vi "DataLog Logging Module.vi"(5 "LuaVIEW reference":T2, 7 "function index":i32) -> (15 "error out":errorcluster)   [LabVIEW 2012]
doc: "Modules required by the \"datalogging\" runlevel. It initializes the logging objects required when the current database goes live. It also exports functions for monitoring and influencing the logging."
uses:
  luaview/typedefs/t_LuaVIEW Reference.ctl
  typedefs/t_DataLog Tag Meta Tags Methods.ctl
  typedefs/t_DataLog Tag Buffers Methods.ctl
  typedefs/t_DataLog Tag Info List Methods.ctl
  typedefs/t_DataLog Live Tag Strings Methods.ctl
  typedefs/t_DataLog Tag Hash Methods.ctl
  typedefs/t_DataLog Aggregation Buffer Methods.ctl
  typedefs/t_DataLog Tag Expression Evaluator Methods.ctl
  luaview/subvis/private/LuaVIEW Pull (string).vi
  luaview/subvis/private/LuaVIEW Pull (refnum).vi
  luaview/subvis/private/LuaVIEW Pull (flat data).vi
  subvis/private/glb_DataLog Runtime Parameterisation.vi
  luaview/subvis/private/LuaVIEW Push (boolean).vi
  luaview/subvis/private/LuaVIEW Push (number).vi
panel:
  in  "config":T1={"aggregation capacity"=100000, "aggregation fraction"=0.7, "min capacity"=64} {"aggregation fraction" format="%.2f"}
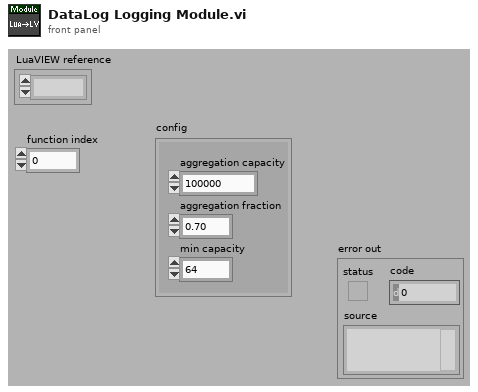
[diagram p1: front panel]
types:
  T1 = cluster{"aggregation capacity":i32, "aggregation fraction":dbl, "min capacity":i32}
  T2 = typedef "t_LuaVIEW Reference.ctl" = refnum<k1>
  T3 = enum32{"initialize", "init objects", "init rebuffer", "init aggregation&recovery", "init error?", "!bool:flushed=flush_next()", "!bool:flushed=flush_next_if()", "!update_recovery()", "!num:size,num:used,num:free=volume_info()", "revoke_exports()", "cleanup()"}
  T4 = typedef "t_DataLog Live Tag Strings Methods.ctl" = enum16{"initialize", "rebuffer", "read", "write", "cleanup"}
  T5 = typedef "t_DataLog Tag Info List Methods.ctl" = enum16{"initialize", "create", "create empty", "rename", "delete", "test tag", "get", "get by name", "get default", "get list", "get path", "get subsets", "set subsets", "set config", "set capacity", "#tags", "go live", "set unlocked", "set mirrored"}
  T6 = typedef "t_DataLog Tag Buffers Methods.ctl" = enum16{"initialize", "inert", "write", "read", "read oldest", "read last", "cleanup"}
  T7 = typedef "t_DataLog Tag Meta Tags Methods.ctl" = enum16{"initialize", "apply and write", "get exceeded", "get metas", "cleanup"}
  T8 = typedef "t_DataLog Tag Hash Methods.ctl" = enum16{"initialize", "add tag", "index tag", "lookup", "#tags", "cleanup", "write recovery", "read recovery", "delete recovery"}
  T9 = typedef "t_DataLog Aggregation Buffer Methods.ctl" = enum16{"initialize", "write", "write special", "flush", "flush next", "flush next if", "setup recovery", "update recovery", "verify recovery", "dummy flush ", "cleanup"}
  T10 = typedef "t_DataLog Tag Expression Evaluator Methods.ctl" = enum16{"set", "get", "eval", "assign", "execute", "isvalid", "clear"}
  T11 = typedef "t_DataLog Tag Config.ctl" = cluster{"name":string, "unit":string, "temporal":T12, "value":T13, "index":i32, "capacity":i32, "is meta?":bool, "mincapacity":i32, "deadband":dbl, "limit delay":dbl, "format":T14, "precision":u8, "undefine":bool, "update":bool, "update period":u16, "expression":string, "description":string, "logging algorithm":T15, "logging parameters":dbl[]}
  T12 = typedef "t_DataLog Temporal Types.ctl" = enum16{"set&hold", "sample", "event"}
  T13 = typedef "t_DataLog Value Types.ctl" = enum16{"number", "string"}
  T14 = typedef "t_DataLog Numerical Format.ctl" = enum8{"fractional", "exponential", "engineering"}
  T15 = typedef "t_DataLog Logging Algorithms.ctl" = enum16{"nothing", "changes", "everything", "every Nth", "time threshold", "value threshold + prior", "t or v threshold", "t or v threshold + prior"}
  T16 = typedef "t_DataLog Point.ctl" = cluster{"time":dbl, "value":dbl}
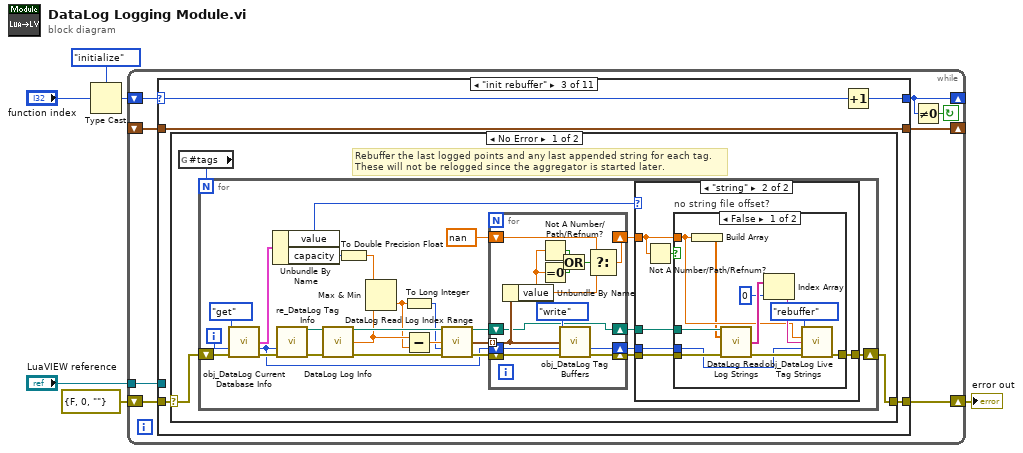
[diagram p0: block diagram]
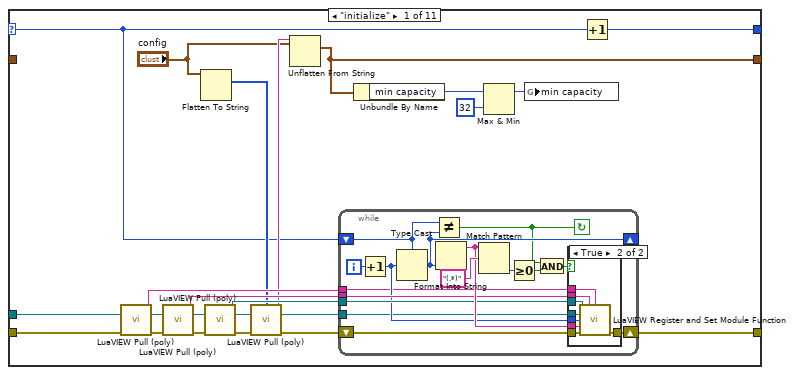
[diagram p2: hidden frame]
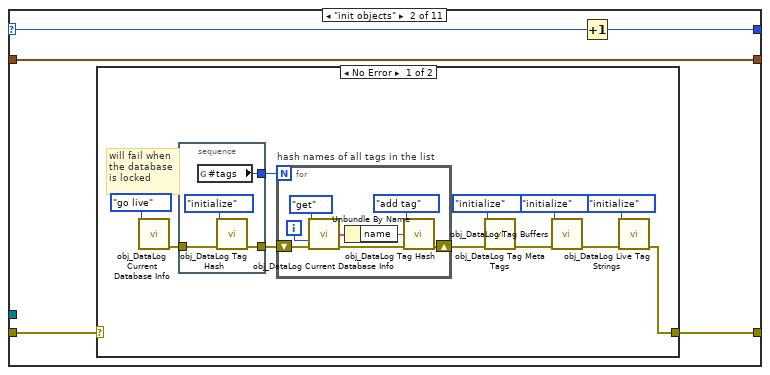
[diagram p4: hidden frame]
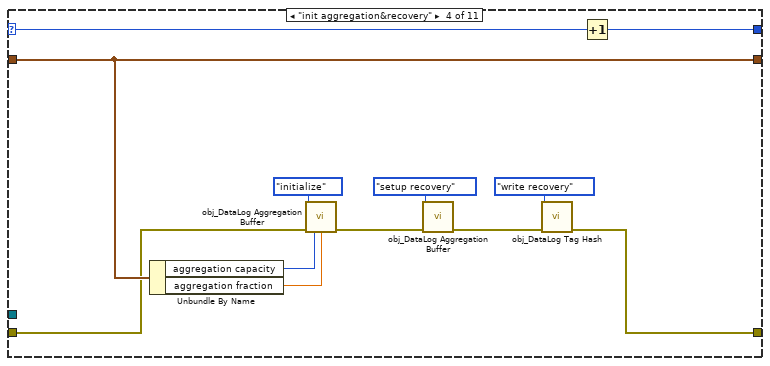
[diagram p9: hidden frame]
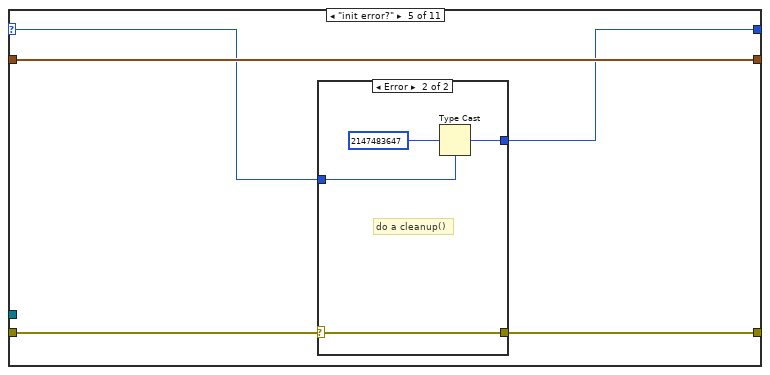
[diagram p10: hidden frame]
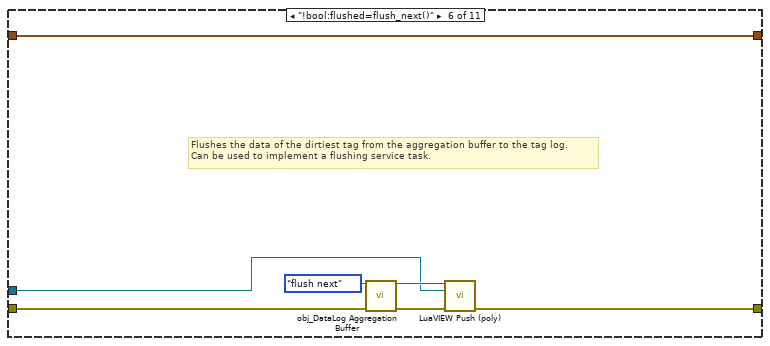
[diagram p12: hidden frame]
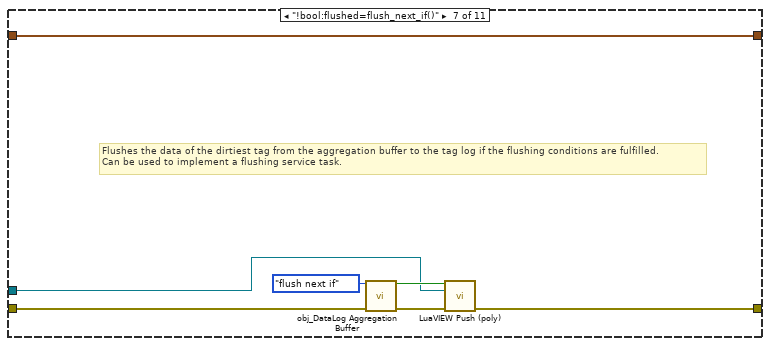
[diagram p13: hidden frame]
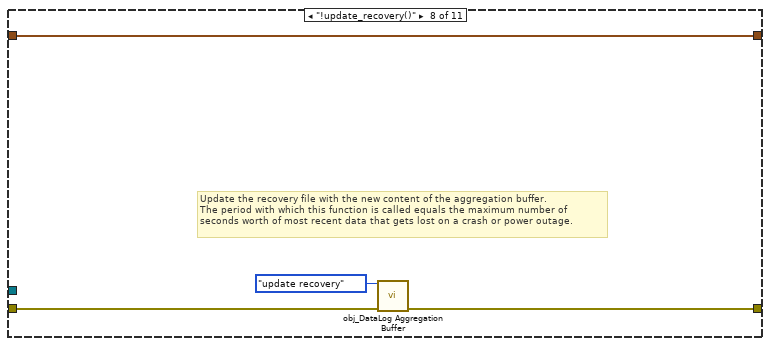
[diagram p14: hidden frame]
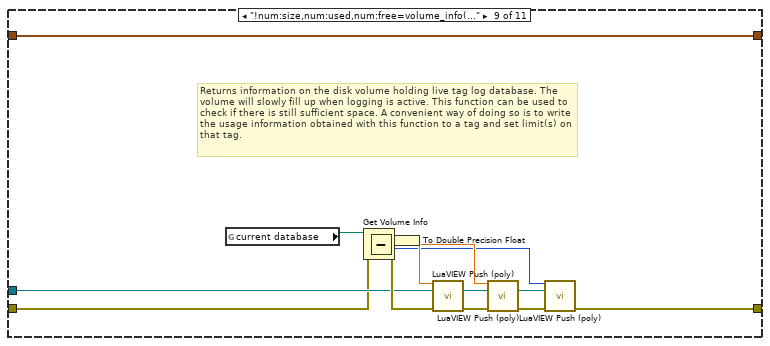
[diagram p15: hidden frame]
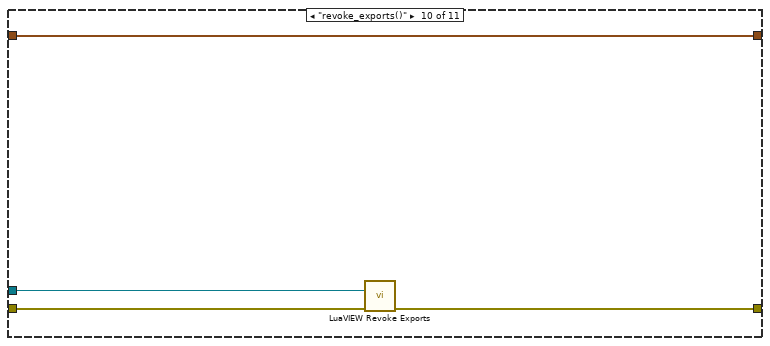
[diagram p16: hidden frame]
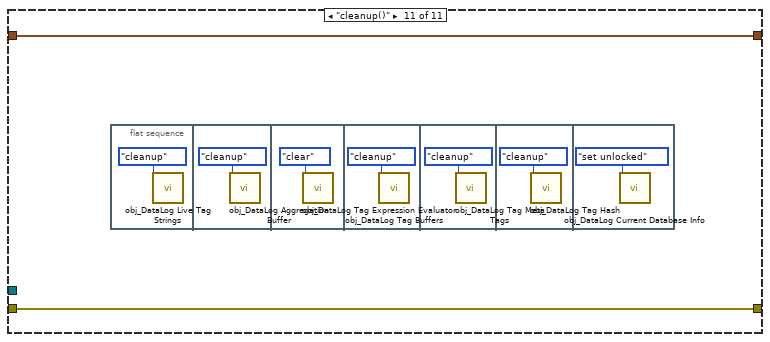
[diagram p17: hidden frame]
diagram:
  n1 = Type Cast(type=T3."initialize" ("cases"), x="function index") -> (*(type *) &x=w5:T3)
  n2 = while {
    shift-right: [w8] -> _
    shift-left: w5 -> [w14]
    shift-right: [w13] -> w6
    shift-left: errorcluster {"status"=FALSE, "code"=0, "source"=""} ("error out") -> [w12]
    shift-right: [w9] -> _
    shift-left: _ -> [w11]
    tunnel: "LuaVIEW reference" -> [w10]
    stop <- w7 continue-if-true
    n3 = case shown="\"init rebuffer\"" w14 {
      selector: w14 -> [w19 w63 w93 w159 w173 _ _ _ _ _ _]
      tunnel: [w20 w64 w92 w160 w172 _ _ _ _ _ _] -> w8
      tunnel: w10 -> [w30 _ _ _ _ w181 w188 _ w202 w213 _]
      tunnel: [w28 w65 w95 w162 w171 w183 w190 w196 w203 w214 w217] -> w13
      tunnel: w12 -> [w29 w66 w94 w161 w174 w182 w189 w195 w201 w215 w217]
      tunnel: w11 -> [_ w67 w96 w163 w175 w187 w194 w198 w212 w216 w218]
      tunnel: [w18 w67 w96 w163 w175 w187 w194 w198 w212 w216 w218] -> w9
      frame "initialize" {
        n4 = call-poly "LuaVIEW Pull (poly).vi"("LuaVIEW reference in"=w30, "error in (no error)"=w29) -> ("string"=w33:string, "LuaVIEW reference out"=w35:T2, "error out"=w34:errorcluster)  [unwired: 11 in]
        n5 = call-poly "LuaVIEW Pull (poly).vi"("LuaVIEW reference in"=w35, "error in (no error)"=w34) -> ("string"=w37:string, "LuaVIEW reference out"=w31:T2, "error out"=w32:errorcluster)  [unwired: 11 in]
        n6 = Flatten To String(anything="config") -> (type string=w22:i16[])  [unwired: 3 in, 2 out]
        n7 = call-poly "LuaVIEW Pull (poly).vi"("LuaVIEW reference in"=w31, "error in (no error)"=w32) -> ("refnum"=w36:refnum<vi>, "LuaVIEW reference out"=w24:T2, "error out"=w27:errorcluster)  [unwired: 11 in]
        n8 = call-poly "LuaVIEW Pull (poly).vi"("type descriptor"=w22, "LuaVIEW reference in"=w24, "error in (no error)"=w27) -> ("flat data"=w23:string, "LuaVIEW reference out"=w25:T2, "error out"=w26:errorcluster)  [unwired: 10 in]
        n9 = Unflatten From String(type="config", binary string=w23) -> (value=w18:T1)  [unwired: 3 in, 2 out]
        n10 = while {
          tunnel: w33 -> [w41]
          shift-right: [w50] -> w28
          shift-left: w26 -> [w51]
          shift-right: [w46] -> _
          shift-left: w19 -> [w47]
          tunnel: w37 -> [w44]
          tunnel: w25 -> [w42]
          tunnel: w36 -> [w45]
          i -> [w49]
          stop <- w38 continue-if-true
          n11 = Increment(x=w49) -> (x+1=w43:i32)
          n12 = Type Cast(type=w47, x=w43) -> (*(type *) &x=w46:T3)
          n13 = Not Equal?(x=w47, y=w46) -> (x != y?=w38:bool)
          n14 = Format Into String(w46) -> (resulting string=w48:string)  [unwired: 3 in, 1 out]
          n15 = Match Pattern(string=w48, regular expression="(.*)") -> (offset past match=w52:i32)  [unwired: 1 in, 3 out]
          n16 = Greater Or Equal To 0?(x=w52) -> (x >= 0?=w40:bool)
          n17 = And(x=w38, y=w40) -> (x .and. y?=w39:bool)
          n18 = case shown="True" w39 {
            tunnel: w41 -> [_ w56]
            tunnel: w42 -> [_ w60]
            tunnel: w43 -> [_ w61]
            tunnel: w48 -> [_ w58]
            tunnel: [w54 w62] -> w50
            tunnel: w51 -> [w54 w59]
            tunnel: w44 -> [_ w57]
            tunnel: w45 -> [_ w55]
            frame False {
            }
            frame True {
              n19 = call "LuaVIEW Register and Set Module Function.vi"("module refnum"=w55, "export table (set as global)"=w57, "table (set as global)"=w56, "LuaVIEW reference in"=w60, "index"=w61, "synopsis"=w58, "error in (no error)"=w59) -> ("error out"=w62:errorcluster)  [unwired: 7 in, 1 out]
            }
          }
        }
        n20 = Unbundle By Name(w18) -> ("min capacity"=w17:i32)
        n21 = Max & Min(x=w17, y=32) -> (max(x,y)=w16:i32)  [unwired: 1 out]
        n22 = global write "glb_DataLog Runtime Parameterisation.vi" "min capacity"(w16) -> ()
        n23 = Increment(x=w19) -> (x+1=w20:T3)
      }
      frame "init objects" {
        n24 = case shown="No Error" w66 {
          selector: w66 -> [_ w91]
          tunnel: [w69 w91] -> w65
          frame No Error {
            # "will fail when\nthe database\nis locked"
            n25 = call "obj_DataLog Current Database Info.vi"("method"=t_DataLog_Tag_Info_List_Methods."go live") -> ("error out"=w71:errorcluster)  [unwired: 8 in, 6 out]
            n26 = stacked-sequence {
              tunnel: [w81] -> w78
              tunnel: [w79] -> w72
              tunnel: w71 -> [w80]
              frame #0 {
                n27 = global read "glb_DataLog Runtime Parameterisation.vi" "#tags"() -> (w79:i32)
                n28 = call "obj_DataLog Tag Hash.vi"("method"=t_DataLog_Tag_Hash_Methods."initialize", "error in (no error)"=w80) -> ("error out"=w81:errorcluster)  [unwired: 10 in, 3 out]
              }
            }
            n29 = for "hash names of all tags in the list" {
              N: w72 -> [_]
              shift-right: [w88] -> w73
              shift-left: w78 -> [w84]
              i -> [w87]
              n30 = call "obj_DataLog Current Database Info.vi"("method"=t_DataLog_Tag_Info_List_Methods."get", "tag index/change#"=w87, "error in (no error)"=w84) -> ("tag config out"=w86:T11, "error out"=w83:errorcluster)  [unwired: 6 in, 5 out]
              n31 = Unbundle By Name(w86) -> ("name"=w85:string)
              n32 = call "obj_DataLog Tag Hash.vi"("method"=t_DataLog_Tag_Hash_Methods."add tag", "tag in"=w85, "error in (no error)"=w83) -> ("error out"=w88:errorcluster)  [unwired: 9 in, 3 out]
            }
            n33 = call "obj_DataLog Tag Meta Tags.vi"("method"=t_DataLog_Tag_Meta_Tags_Methods."initialize", "error in (no error)"=w73) -> ("error out"=w74:errorcluster)  [unwired: 9 in, 4 out]
            n34 = call "obj_DataLog Tag Buffers.vi"("method"=t_DataLog_Tag_Buffers_Methods."initialize", "error in (no error)"=w74) -> ("error out"=w70:errorcluster)  [unwired: 9 in, 4 out]
            n35 = call "obj_DataLog Live Tag Strings.vi"("method"=t_DataLog_Live_Tag_Strings_Methods."initialize", "error in (no error)"=w70) -> ("error out"=w69:errorcluster)  [unwired: 10 in, 3 out]
          }
          frame Error {
          }
        }
        n36 = Increment(x=w63) -> (x+1=w64:T3)
      }
      frame "init rebuffer" {
        n37 = case shown="No Error" w94 {
          selector: w94 -> [w99 w158]
          tunnel: [w98 w158] -> w95
          frame No Error {
            # "Rebuffer the last logged points and any last appended string for each tag.\nThese will not be relogged since the aggregator is started later."
            n38 = global read "glb_DataLog Runtime Parameterisation.vi" "#tags"() -> (w97:i32)
            n39 = for {
              N: w97 -> [_]
              shift-right: [w106] -> w98
              shift-left: w99 -> [w122]
              i -> [w123]
              n40 = call "obj_DataLog Current Database Info.vi"("method"=t_DataLog_Tag_Info_List_Methods."get", "tag index/change#"=w123, "error in (no error)"=w122) -> ("tag config out"=w124:T11, "dup tag index"=w100:i32, "error out"=w121:errorcluster)  [unwired: 6 in, 4 out]
              n41 = Unbundle By Name(w124) -> ("value"=w107:T13, "capacity"=w113:i32)
              n42 = call "re_DataLog Tag Info.vi"("tag index (use tag)"=w100, "error in (no error)"=w121) -> ("tag log directory"=w118:path, "error out"=w119:errorcluster)  [unwired: 10 in, 2 out]
              n43 = call "DataLog Log Info.vi"("tag log directory"=w118, "error in (no error)"=w119) -> ("dup tag log directory"=w117:path, "size"=w111:dbl, "error out"=w120:errorcluster)  [unwired: 10 in, 1 out]
              n44 = To Double Precision Float(number=w113) -> (double precision float=w112:dbl)
              n45 = Max & Min(x=w112, y=w111) -> (min(x,y)=w110:dbl)  [unwired: 1 out]
              n46 = To Long Integer(number=w110) -> (32bit integer=w109:i32)
              n47 = Subtract(x=w111, y=w110) -> (x-y=w114:dbl)
              n48 = call "DataLog Read Log Index Range.vi"("tag log directory"=w117, "log index"=w114, "number of points"=w109, "error in (no error)"=w120) -> ("dup tag log directory"=w103:path, "range of points"=w115:T16[], "error out"=w116:errorcluster)  [unwired: 9 in]
              n49 = for {
                shift-right: [w157] -> w105
                shift-left: w116 -> [w155]
                tunnel: w115 -> [w154] mode=indexing
                shift-right: [w148] -> w104
                shift-left: nan -> [w150]
                shift-right: [w146] -> w102
                shift-left: w100 -> [w147]
                shift-right: [w145] -> w101
                shift-left: w103 -> [w145]
                n50 = Unbundle By Name(w154) -> ("value"=w149:dbl)
                n51 = Not A Number/Path/Refnum?(number/path/refnum=w149) -> (NaN/Path/Refnum?=w153:bool)
                n52 = Equal To 0?(x=w149) -> (x = 0?=w152:bool)
                n53 = Or(x=w153, y=w152) -> (x .or. y?=w151:bool)
                n54 = call "obj_DataLog Tag Buffers.vi"("method"=t_DataLog_Tag_Buffers_Methods."write", "point in"=w154, "tag index"=w147, "error in (no error)"=w155) -> ("tag index dup"=w146:i32, "error out"=w157:errorcluster)  [unwired: 7 in, 3 out]
                n55 = Select(t=w150, s=w151, f=w149) -> (s? t:f=w148:dbl)
              }
              n56 = case shown="\"string\"" w107 {
                tunnel: [w126 w130] -> w106
                tunnel: w105 -> [w126 w131]
                tunnel: w104 -> [_ w129]
                tunnel: w102 -> [_ w128]
                tunnel: w101 -> [_ w127]
                frame "number" {
                }
                frame "string" {
                  n57 = Not A Number/Path/Refnum?(number/path/refnum=w129) -> (NaN/Path/Refnum?=w132:bool)
                  n58 = case "no string file offset?" shown="False" w132 {
                    tunnel: w131 -> [w143 w144]
                    tunnel: [w137 w144] -> w130
                    tunnel: w129 -> [w134 _]
                    tunnel: w128 -> [w138 _]
                    tunnel: w127 -> [w142 _]
                    frame False {
                      n59 = Build Array(w134) -> (w133:dbl[])
                      n60 = call "DataLog Read Log Strings.vi"("tag log directory"=w142, "offsets (use points)"=w133, "error in (no error)"=w143) -> ("strings"=w141:string[], "error out"=w139:errorcluster)  [unwired: 9 in, 2 out]
                      n61 = Index Array(array=w141, index=0) -> (element=w136:string)
                      n62 = call "obj_DataLog Live Tag Strings.vi"("method"=t_DataLog_Live_Tag_Strings_Methods."rebuffer", "offset/time"=w134, "string in"=w136, "tag index"=w138, "error in (no error)"=w139) -> ("error out"=w137:errorcluster)  [unwired: 7 in, 3 out]
                    }
                    frame True {
                    }
                  }
                }
              }
            }
          }
          frame Error {
          }
        }
        n63 = Increment(x=w93) -> (x+1=w92:T3)
      }
      frame "init aggregation&recovery" {
        n64 = Unbundle By Name(w163) -> ("aggregation capacity"=w165:i32, "aggregation fraction"=w164:dbl)
        n65 = call "obj_DataLog Aggregation Buffer.vi"("method"=t_DataLog_Aggregation_Buffer_Methods."initialize", "error in (no error)"=w161, "aggregation capacity {initialize}"=w165, "aggregation fraction {initialize}"=w164) -> ("error out"=w168:errorcluster)  [unwired: 10 in, 1 out]
        n66 = call "obj_DataLog Aggregation Buffer.vi"("method"=t_DataLog_Aggregation_Buffer_Methods."setup recovery", "error in (no error)"=w168) -> ("error out"=w166:errorcluster)  [unwired: 12 in, 1 out]
        n67 = call "obj_DataLog Tag Hash.vi"("method"=t_DataLog_Tag_Hash_Methods."write recovery", "error in (no error)"=w166) -> ("error out"=w162:errorcluster)  [unwired: 10 in, 3 out]
        n68 = Increment(x=w159) -> (x+1=w160:T3)
      }
      frame "init error?" {
        n69 = case shown="Error" w174 {
          selector: w174 -> [w176 w178]
          tunnel: w173 -> [_ w179]
          tunnel: [w176 w178] -> w171
          tunnel: [_ w177] -> w172
          frame No Error {
          }
          frame Error {
            # "do a cleanup()"
            n70 = Type Cast(type=w179, x=2147483647) -> (*(type *) &x=w177:T3)
          }
        }
      }
      frame "!bool:flushed=flush_next()" {
        # "Flushes the data of the dirtiest tag from the aggregation buffer to the tag log.\nCan be used to implement a flushing service task."
        n71 = call "obj_DataLog Aggregation Buffer.vi"("method"=t_DataLog_Aggregation_Buffer_Methods."flush next", "error in (no error)"=w182) -> ("flush needed?"=w184:bool, "error out"=w185:errorcluster)  [unwired: 12 in]
        n72 = call-poly "LuaVIEW Push (poly).vi"("boolean"=w184, "LuaVIEW reference in"=w181, "error in (no error)"=w185) -> ("error out"=w183:errorcluster)  [unwired: 11 in, 1 out]
      }
      frame "!bool:flushed=flush_next_if()" {
        # "Flushes the data of the dirtiest tag from the aggregation buffer to the tag log if the flushing conditions are fulfilled.\nCan be used to implement a flushing service task."
        n73 = call "obj_DataLog Aggregation Buffer.vi"("method"=t_DataLog_Aggregation_Buffer_Methods."flush next if", "error in (no error)"=w189) -> ("flush needed?"=w191:bool, "error out"=w192:errorcluster)  [unwired: 12 in]
        n74 = call-poly "LuaVIEW Push (poly).vi"("boolean"=w191, "LuaVIEW reference in"=w188, "error in (no error)"=w192) -> ("error out"=w190:errorcluster)  [unwired: 11 in, 1 out]
      }
      frame "!update_recovery()" {
        # "Update the recovery file with the new content of the aggregation buffer.\nThe period with which this function is called equals the maximum number of\nseconds worth of most recent data that gets lost on a crash or power outage."
        n75 = call "obj_DataLog Aggregation Buffer.vi"("method"=t_DataLog_Aggregation_Buffer_Methods."update recovery", "error in (no error)"=w195) -> ("error out"=w196:errorcluster)  [unwired: 12 in, 1 out]
      }
      frame "!num:size,num:used,num:free=volume_info()" {
        # "Returns information on the disk volume holding live tag log database. The volume will slowly fill up when logging is active. This function can be used to check if there is still sufficient space. A convenient way of doing so is to write the usage information obtained with this function to a tag and set limit(s) on that tag."
        n76 = global read "glb_DataLog Runtime Parameterisation.vi" "current database"() -> (w200:path)
        n77 = Get Volume Info(8:w201, 11:w200) -> (0:w204:errorcluster, 1:w207:i64, 2:w199:i64)  [unwired: 3 out]
        n78 = To Double Precision Float(number=w199) -> (double precision float=w209:dbl)
        n79 = Subtract(x=w209, y=w207) -> (x-y=w208:dbl)
        n80 = call-poly "LuaVIEW Push (poly).vi"("number"=w209, "LuaVIEW reference in"=w202, "error in (no error)"=w204) -> ("LuaVIEW reference out"=w211:T2, "error out"=w205:errorcluster)  [unwired: 11 in]
        n81 = call-poly "LuaVIEW Push (poly).vi"("number"=w208, "LuaVIEW reference in"=w211, "error in (no error)"=w205) -> ("LuaVIEW reference out"=w210:T2, "error out"=w206:errorcluster)  [unwired: 11 in]
        n82 = call-poly "LuaVIEW Push (poly).vi"("number"=w207, "LuaVIEW reference in"=w210, "error in (no error)"=w206) -> ("error out"=w203:errorcluster)  [unwired: 11 in, 1 out]
      }
      frame "revoke_exports()" {
        n83 = call "LuaVIEW Revoke Exports.vi"("LuaVIEW reference in"=w213, "error in (no error)"=w215) -> ("error out"=w214:errorcluster)  [unwired: 12 in, 1 out]
      }
      frame "cleanup()" {
        n84 = flat-sequence {
          frame #0 {
            n85 = call "obj_DataLog Live Tag Strings.vi"("method"=t_DataLog_Live_Tag_Strings_Methods."cleanup") -> ()  [unwired: 11 in, 4 out]
          }
          frame #1 {
            n86 = call "obj_DataLog Aggregation Buffer.vi"("method"=t_DataLog_Aggregation_Buffer_Methods."cleanup") -> ()  [unwired: 13 in, 2 out]
          }
          frame #2 {
            n87 = call "obj_DataLog Tag Expression Evaluator.vi"("method"=t_DataLog_Tag_Expression_Evaluator_Methods."clear") -> ()  [unwired: 13 in, 2 out]
          }
          frame #3 {
            n88 = call "obj_DataLog Tag Buffers.vi"("method"=t_DataLog_Tag_Buffers_Methods."cleanup") -> ()  [unwired: 10 in, 5 out]
          }
          frame #4 {
            n89 = call "obj_DataLog Tag Meta Tags.vi"("method"=t_DataLog_Tag_Meta_Tags_Methods."cleanup") -> ()  [unwired: 10 in, 5 out]
          }
          frame #5 {
            n90 = call "obj_DataLog Tag Hash.vi"("method"=t_DataLog_Tag_Hash_Methods."cleanup") -> ()  [unwired: 11 in, 4 out]
          }
          frame #6 {
            n91 = call "obj_DataLog Current Database Info.vi"("method"=t_DataLog_Tag_Info_List_Methods."set unlocked") -> ()  [unwired: 8 in, 7 out]
          }
        }
      }
    }
    n92 = Not Equal To 0?(x=w8) -> (x != 0?=w7:bool)
  }
  "error out" <- w6
